vi "Point Turn.vi"(8 "right motors":string="RobotDrive", 9 "Speed":dbl, 10 "Angle":dbl, 11 "left motors":string="RobotDrive") -> ()   [LabVIEW 2019]
uses:
  <vilib>/Rock Robotics/WPI/Utilities/WPI_GetSetVariantRefNum.vi
panel:
  in  "Gyro":string="My ADIS16448 RefNum"
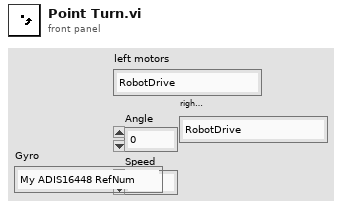
[diagram p1: front panel]
types:
  T1 = typedef "ADIS16448 Device Reference.ctl" = cluster{"DevStatus":errorcluster, "Hardware Config":T2, "Calibration Complete":refnum<notifier>, "Status FIFO":refnum<k33>, "Last Value Reference":refnum<data-value>, "Sychronous Process VI":T6, "Cmd FIFO":refnum<k33>, "Source":T7, "Data FIFO":refnum<k33>, "IMU Status LED Pin":T4, "Calibration Time":u32}
  T2 = typedef "ADIS16448 Hardware Configuration.ctl" = cluster{"SPI Clock Rate (Hz)":dbl, "IMU SPI Mode (3)":T3, "IMU Reset Pin":T4, "IMU SPI Bus":T5, "IMU Data Ready Pin":T4, "Stall Config":cluster{"Pow2BytesPerRead":u8, "StallTicks":u16, "CsToSclkTicks":u8}, "IMU Status LED Pin":T4}
  T3 = typedef "WPI_SPIMode.ctl" = enum16{"Mode 0 (Clk Idle Low,Sample on Leading)", "Mode 1 (Clk Idle Low,Sample on Trailing)", "Mode 2 (Clk Idle High,Sample on Leading)", "Mode 3 (Clk Idle High,Sample on Trailing)"}
  T4 = typedef "FPGA_DIOChannel.ctl" = enum8{"DIO 0", "DIO 1", "DIO 2", "DIO 3", "DIO 4", "DIO 5", "DIO 6", "DIO 7", "DIO 8", "DIO 9", "DIO MXP 0", "DIO MXP 1", "DIO MXP 2", "DIO MXP 3", "DIO MXP 4", "DIO MXP 5", "DIO MXP 6", "DIO MXP 7", "DIO MXP 8", "DIO MXP 9", "DIO MXP 10", "DIO MXP 11", "DIO MXP 12", "DIO MXP 13", "DIO MXP 14", "DIO MXP 15", "SPI Port CS1", "SPI Port CS2", "SPI Port CS3", "SPI Port MISO", "SPI Port MOSI", "Invalid"}
  T5 = typedef "spi_bus.ctl" = enum16{"SPI On-Board, CS0", "SPI On-Board, CS1", "SPI On-Board, CS2", "SPI On-Board, CS3", "SPI MXP", "Invalid"}
  T6 = typedef "ADIS16448 Process.ctl" = refnum<vi>
  T7 = typedef "FPGA_CounterEncoderSourceConvertionLVSourceType.ctl" = cluster{"DevStatus":errorcluster, "AnalogTriggerMode?":bool, "DigitalMode":cluster{"DIO Channel":T8}, "AnalogTriggerMode":cluster{"AnalogTriggerIndex":T9, "OutputType":T10}}
  T8 = typedef "FPGA_DIODigitalSourceChannel.ctl" = enum8{"DIO 0", "DIO 1", "DIO 2", "DIO 3", "DIO 4", "DIO 5", "DIO 6", "DIO 7", "DIO 8", "DIO 9", "DIO MXP 0", "DIO MXP 1", "DIO MXP 2", "DIO MXP 3", "DIO MXP 4", "DIO MXP 5", "DIO MXP 6", "DIO MXP 7", "DIO MXP 8", "DIO MXP 9", "DIO MXP 10", "DIO MXP 11", "DIO MXP 12", "DIO MXP 13", "DIO MXP 14", "DIO MXP 15", "SPI Port CS1", "SPI Port CS2", "SPI Port CS3", "SPI Port MISO", "SPI Port MOSI", "Disabled"}
  T9 = typedef "FPGA_AnalogTriggerIndex.ctl" = enum8{"Trig 0", "Trig 1", "Trig 2", "Trig 3", "Trig 4", "Trig 5", "Trig 6", "Trig 7", "Invalid"}
  T10 = typedef "FPGA_AnalogTriggerOutType.ctl" = enum16{"InWindow", "TriggerState", "Rising", "Falling"}
  T11 = typedef "ADIS16448 Data.ctl" = cluster{"XAngle":dbl, "YAngle":dbl, "ZAngle":dbl}
  T12 = typedef "WPI_RobotDriveDevRef.ctl" = cluster{"DevStatus":errorcluster, "Motors[]":T13[], "Square Inputs":bool, "Max Output":dbl}
  T13 = typedef "WPI_MotorControlDeviceRef.ctl" = cluster{"DeviceStatus":errorcluster, "Type":T14, "PWM":cluster{"PWM Channel":T15, "DeadBand":T16}, "CAN":cluster{"Device Number":u8, "SetOutput VI Ref":variant, "GetOutput VI Ref":variant, "Enable VI Ref":variant, "Disable VI Ref":variant, "Data":variant}, "Invert":bool, "DIO PWM":cluster{"PWM \"Enable\" Channel":T15, "DIOChannel":T4, "PWM Rate":dbl}}
  T14 = typedef "WPI_MotorControlType.ctl" = enum16{"PWM", "CAN", "DIO PWM"}
  T15 = typedef "FPGA_DIOPWMChannel.ctl" = enum8{"PWM 0", "PWM 1", "PWM 2", "PWM 3", "PWM 4", "PWM 5", "PWM 6", "PWM 7", "PWM 8", "PWM 9", "PWM MXP 0", "PWM MXP 1", "PWM MXP 2", "PWM MXP 3", "PWM MXP 4", "PWM MXP 5", "PWM MXP 6", "PWM MXP 7", "PWM MXP 8", "PWM MXP 9", "Invalid"}
  T16 = typedef "WPI_PWMDeadband.ctl" = cluster{"Name":string, "maxPositivePwm":i32, "minPositivePwm":i32, "centerPwm":i32, "maxNegativePwm":i32, "minNegativePwm":i32, "angularRange":u16}
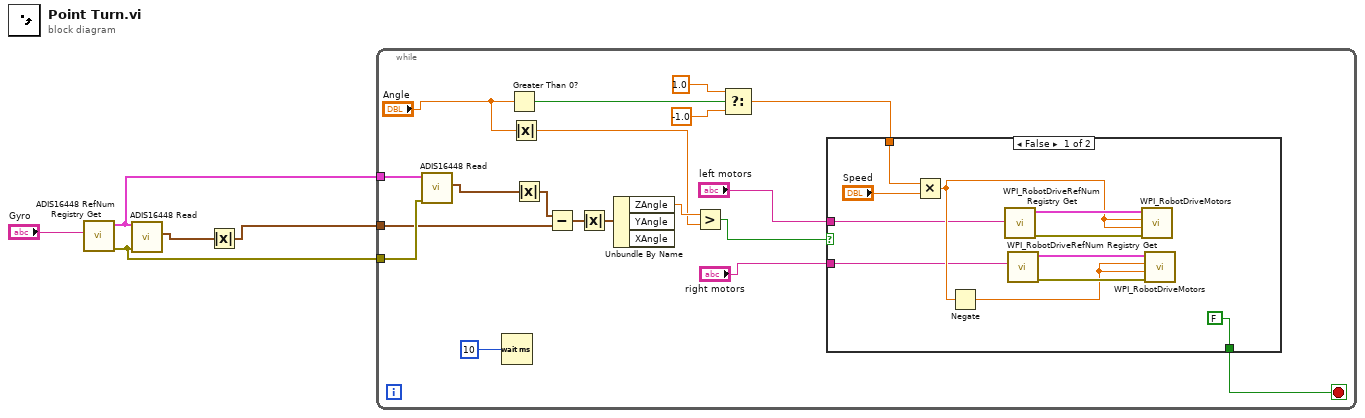
[diagram p0: block diagram]
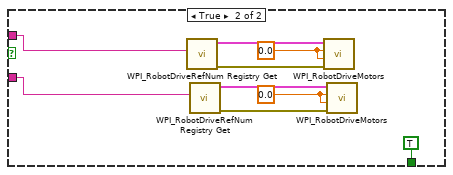
[diagram p2: hidden frame]
diagram:
  n1 = call <vilib>:"ADIS16448 RefNum Registry Get.vi"("refnum name"="Gyro") -> ("error out"=w3:errorcluster, "ADIS16448DevRef Out"=w4:T1)  [unwired: 9 in]
  n2 = call <vilib>:"ADIS16448 Read.vi"("error in (no error)"=w3, "ADIS16448DevRef"=w4) -> ("ADIS16448 Value"=w2:T11)  [unwired: 6 in, 3 out]
  n3 = Absolute Value(x=w2) -> (abs(x)=w1:T11)
  n4 = while {
    tunnel: w4 -> [w18]
    tunnel: w3 -> [w17]
    tunnel: w1 -> [w12]
    stop <- w19 stop-if-true
    n5 = call <vilib>:"ADIS16448 Read.vi"("error in (no error)"=w17, "ADIS16448DevRef"=w18) -> ("ADIS16448 Value"=w14:T11)  [unwired: 6 in, 3 out]
    n6 = Wait (ms)(milliseconds to wait=u32 10 ("millisecond timer value")) -> ()  [unwired: 1 out]
    n7 = Greater Than 0?(x="Angle") -> (x > 0?=w24:bool)
    n8 = Absolute Value(x="Angle") -> (abs(x)=w7:dbl)
    n9 = Absolute Value(x=w14) -> (abs(x)=w13:T11)
    n10 = Subtract(x=w13, y=w12) -> (x-y=w11:T11)
    n11 = Absolute Value(x=w11) -> (abs(x)=w10:T11)
    n12 = Unbundle By Name(w10) -> ("ZAngle"=w9:dbl)  [unwired: 2 out]
    n13 = Greater?(x=w9, y=w7) -> (0:w6:bool)
    n14 = Select(t=1.0, s=w24, f=-1.0) -> (s? t:f=w21:dbl)
    n15 = case shown="False" w6 {
      tunnel: w21 -> [w31 _]
      tunnel: [FALSE TRUE] -> w19
      tunnel: "left motors" -> [w26 w37]
      tunnel: "right motors" -> [w25 w36]
      frame False {
        n16 = Multiply(x=w31, y="Speed") -> (x*y=w28:dbl)
        n17 = Negate(x=w28) -> (-x=w29:dbl)
        n18 = call <vilib>:"WPI_RobotDriveRefNum Registry Get.vi"("refnum name"=w26) -> ("error out"=w33:errorcluster, "RobotDriveDevRef"=w32:T12)  [unwired: 9 in]
        n19 = call <vilib>:"WPI_RobotDriveRefNum Registry Get.vi"("refnum name"=w25) -> ("error out"=w35:errorcluster, "RobotDriveDevRef"=w34:T12)  [unwired: 9 in]
        n20 = call <vilib>:"WPI_RobotDriveMotors.vi"("error in (no error)"=w33, "RightSpeed"=w28, "LeftSpeed"=w28, "RobotDriveDevRef"=w32) -> ()  [unwired: 5 in, 3 out]
        n21 = call <vilib>:"WPI_RobotDriveMotors.vi"("error in (no error)"=w35, "RightSpeed"=w29, "LeftSpeed"=w29, "RobotDriveDevRef"=w34) -> ()  [unwired: 5 in, 3 out]
      }
      frame True {
        w40 = 0.0 ("LeftSpeed")
        w41 = 0.0 ("LeftSpeed")
        n22 = call <vilib>:"WPI_RobotDriveRefNum Registry Get.vi"("refnum name"=w37) -> ("error out"=w43:errorcluster, "RobotDriveDevRef"=w44:T12)  [unwired: 9 in]
        n23 = call <vilib>:"WPI_RobotDriveRefNum Registry Get.vi"("refnum name"=w36) -> ("error out"=w39:errorcluster, "RobotDriveDevRef"=w42:T12)  [unwired: 9 in]
        n24 = call <vilib>:"WPI_RobotDriveMotors.vi"("error in (no error)"=w43, "RightSpeed"=w41, "LeftSpeed"=w41, "RobotDriveDevRef"=w44) -> ()  [unwired: 5 in, 3 out]
        n25 = call <vilib>:"WPI_RobotDriveMotors.vi"("error in (no error)"=w39, "RightSpeed"=w40, "LeftSpeed"=w40, "RobotDriveDevRef"=w42) -> ()  [unwired: 5 in, 3 out]
      }
    }
  }
